vi "Terminate.vi"(8 "error in (no error)":errorcluster, 10 "Message in":refnum<class "TerminateMessage.lvclass">, 11 "StageSPIM in":refnum<class "StageSPIM.lvclass">) -> (0 "error out":errorcluster, 3 "StageSPIM out":refnum<class "StageSPIM.lvclass">)   [LabVIEW 2012, in "StageSPIM.lvclass"]
doc: "This member function is called when the statemachine in the run.vi receives an 'terminate' command. It closes the RabbitMQ connection. \n\nOverride this member function in your derived class to release all previously acquired resources (but don't forget to call the parent method). If your component has subcomponents, they count as resources, and you have to release them by calling their own terminate functions."
uses:
  StageSPIM.lvclass
  <vilib>/Distrio/Murmex/TerminateMessage/TerminateMessage.lvclass
  <vilib>/Distrio/Murmex/Murmex/Murmex.lvclass
panel:
  out "Array":bool[](array[boolean])
  # "This method is called when the TERMINATE\ntrigger is sent. \n\nOverride this method when your component needs to\nrespond to this trigger. \n\nCall parent for proper implementation"
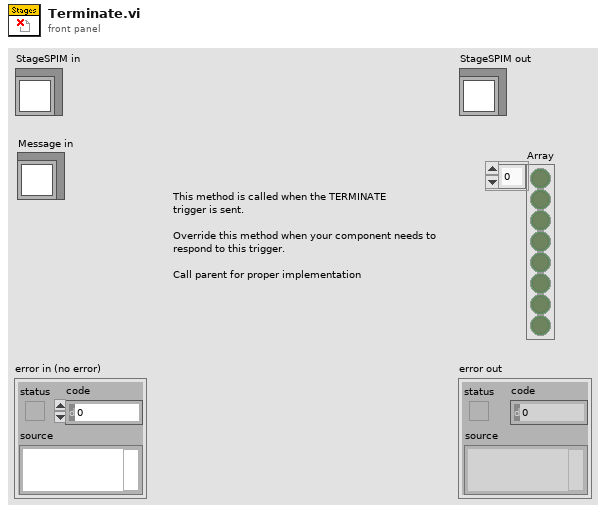
[diagram p1: front panel]
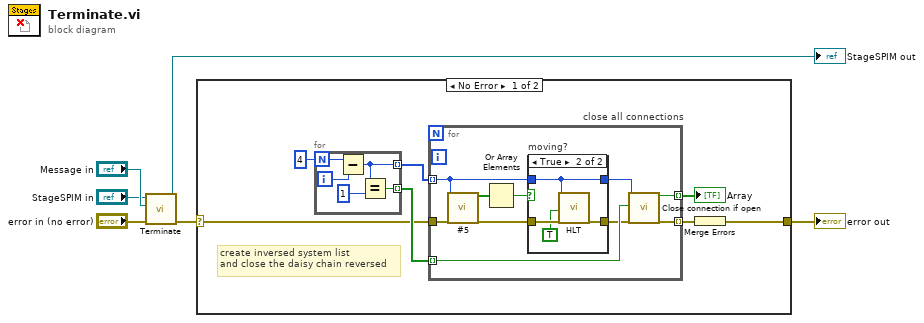
[diagram p0: block diagram]
diagram:
  n1 = call-parent "Terminate.vi"("error in (no error)"="error in (no error)", "Message in"="Message in", "Murmex in"="StageSPIM in") -> ("error out"=w3:errorcluster, "Murmex out"=→"StageSPIM out":refnum<class "StageSPIM.lvclass">)  [unwired: 7 in]
  n2 = case shown="No Error" w3 {
    selector: w3 -> [w8 w35]
    tunnel: [w7 w35] -> w2
    frame No Error {
      # "create inversed system list\nand close the daisy chain reversed"
      n3 = for {
        N: 4 -> [w18]
        tunnel: [w16] -> w11 mode=indexing
        tunnel: [w14] -> w10 mode=indexing
        i -> [w17]
        n4 = Subtract(x=w18, y=w17) -> (x-y=w16:i32)
        n5 = Equal?(x=w16, y=1) -> (x = y?=w14:bool)
      }
      n6 = for "close all connections" {
        tunnel: w11 -> [w24] mode=indexing
        tunnel: w10 -> [w28] mode=indexing
        tunnel: [w27] -> w13 mode=indexing
        tunnel: w8 -> [w23]
        tunnel: [w26] -> w12 mode=indexing
        n7 = call "#5.vi"("System no."=w24, "error in"=w23) -> ("Axis moving?"=w21:bool[], "error out"=w22:errorcluster)  [unwired: 16 in]
        n8 = Or Array Elements(Boolean array=w21) -> (logical OR=w20:bool)
        n9 = case "moving?" shown="True" w20 {
          tunnel: [w29 w34] -> w25
          tunnel: w24 -> [w30 w31]
          tunnel: w22 -> [w29 w33]
          tunnel: [w30 w31] -> w19
          frame False {
          }
          frame True {
            n10 = call "HLT.vi"("System no."=w31, "All axes?"=TRUE ("all axes"), "error in"=w33) -> ("error out"=w34:errorcluster)  [unwired: 16 in]
          }
        }
        n11 = call "Close connection if open.vi"("System no."=w19, "Close DaisyChain"=w28, "error in"=w25) -> ("Was connected?"=w27:bool, "error out"=w26:errorcluster)  [unwired: 15 in]
      }
      "Array" <- w13
      n12 = Merge Errors(w12) -> (w7:errorcluster)
    }
    frame Error {
    }
  }
  "error out" <- w2
